vi "Calling VI Ref If Not Valid.vi"(4 "Chain Index":i32=-1, 6 "Open Relationship (Caller)":T1(ring), 8 "error in (no error)":errorcluster, 9 "VI Reference":refnum<vi>) -> (0 "error out":errorcluster, 1 "Valid VI Ref":refnum<vi>, 2 "New Reference Opened":bool)   [LabVIEW 2011]
doc: "This VI will make a <B>Valid VI Ref</B> if the <B>VI Reference</B> being passed in is not valid. It does this by opening a reference to a VI in the chain. By default the calling VI will be opened but this can be changed with the enum <B>Open Relationship (Caller)</B> or the <B>Chain Index</B> controls.\n\n-------------\nDeveloped by Brian Hoover (hooovahh)"
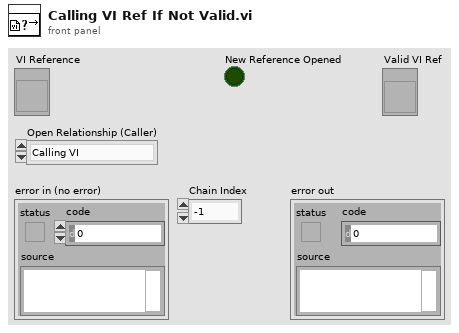
[diagram p1: front panel]
types:
  T1 = enum16{"Calling VI", "Callers Caller", "Callers Callers Caller"}
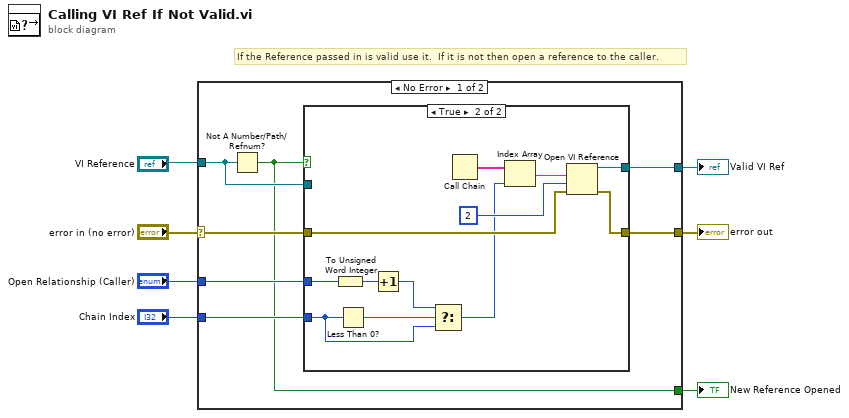
[diagram p0: block diagram]
diagram:
  # "If the Reference passed in is valid use it.  If it is not then open a reference to the caller."
  n1 = case shown="No Error" "error in (no error)" {
    selector: "error in (no error)" -> [w9 w30]
    tunnel: "VI Reference" -> [w14 w29]
    tunnel: [w13 w29] -> w6
    tunnel: [w12 w30] -> w5
    tunnel: "Open Relationship (Caller)" -> [w11 _]
    tunnel: "Chain Index" -> [w10 _]
    tunnel: [w8 _] -> w1
    frame No Error {
      n2 = Not A Number/Path/Refnum?(number/path/refnum=w14) -> (NaN/Path/Refnum?=w8:bool)
      n3 = case shown="True" w8 {
        tunnel: w14 -> [w16 _]
        tunnel: [w16 w25] -> w13
        tunnel: w9 -> [w15 w24]
        tunnel: [w15 w23] -> w12
        tunnel: w11 -> [_ w20]
        tunnel: w10 -> [_ w21]
        frame False {
        }
        frame True {
          n4 = To Unsigned Word Integer(number=w20) -> (unsigned 16bit integer=w19:u16)
          n5 = Less Than 0?(x=w21) -> (x < 0?=w22:bool)
          n6 = Increment(x=w19) -> (x+1=w18:u16)
          n7 = Select(t=w18, s=w22, f=w21) -> (s? t:f=w17:i32)
          n8 = Call Chain() -> (call chain=w28:string[])
          n9 = Index Array(array=w28, index=w17) -> (element=w27:string)
          n10 = Open VI Reference(vi path=w27, options=2, error in (no error)=w24) -> (vi reference=w25:refnum<vi>, error out=w23:errorcluster)  [unwired: 3 in]
        }
      }
    }
    frame Error {
    }
  }
  "Valid VI Ref" <- w6
  "error out" <- w5
  "New Reference Opened" <- w1
